vi "Velocity Acceleration.vi"() -> ()   [LabVIEW 2024]
panel:
  out "String":string
  out "Acceleration":dbl[](array[numeric])
  out "Velocity":dbl[](array[numeric])
  in  "DIsplacement":dbl[](array[numeric])
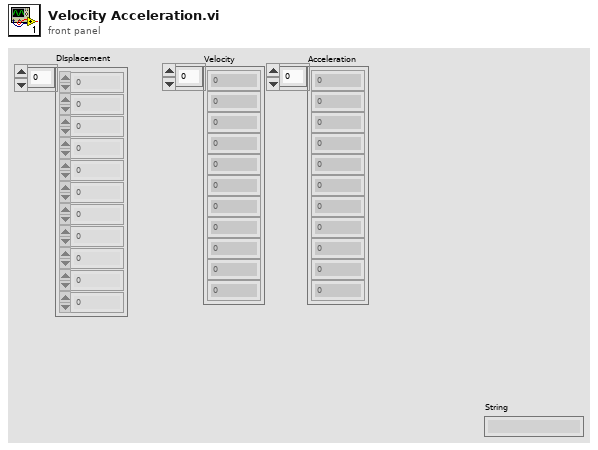
[diagram p1: front panel]
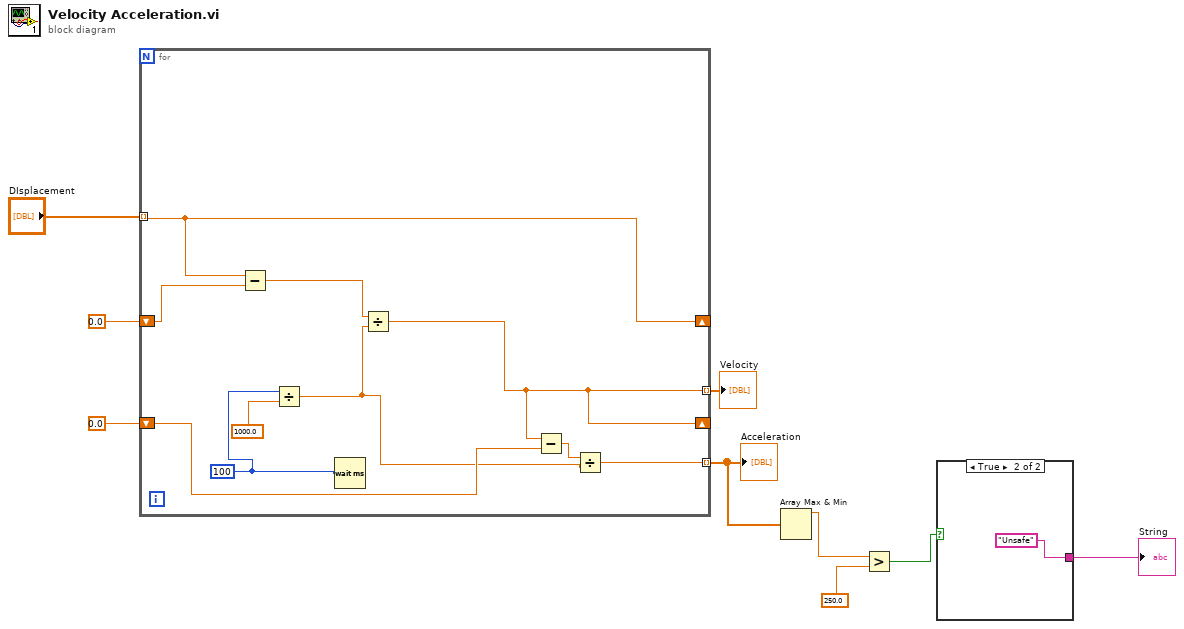
[diagram p0: block diagram]
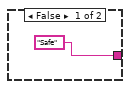
[diagram p2: hidden frame]
diagram:
  n1 = for {
    tunnel: "DIsplacement" -> [w17] mode=indexing
    shift-right: [w17] -> _
    shift-left: 0.0 ("Numeric") -> [w16]
    tunnel: [w13] -> w7 mode=indexing
    shift-right: [w13] -> _
    shift-left: 0.0 -> [w14]
    tunnel: [w10] -> w5 mode=indexing
    w18 = u32 100 ("milliseconds to wait")
    n2 = Subtract(x=w17, y=w16) -> (x-y=w15:dbl)
    n3 = Divide(x=w18, y=1000.0) -> (x/y=w11:dbl)
    n4 = Wait (ms)(milliseconds to wait=w18) -> ()  [unwired: 1 out]
    n5 = Divide(x=w15, y=w11) -> (x/y=w13:dbl)
    n6 = Subtract(x=w13, y=w14) -> (x-y=w12:dbl)
    n7 = Divide(x=w12, y=w11) -> (x/y=w10:dbl)
  }
  "Velocity" <- w7
  "Acceleration" <- w5
  n8 = Array Max & Min(array=w5) -> (max value=w3:dbl)  [unwired: 3 out]
  n9 = Greater?(x=w3, y=250.0) -> (0:w1:bool)
  n10 = case shown="True" w1 {
    tunnel: ["Safe" "Unsafe"] -> w2
    frame False {
    }
    frame True {
    }
  }
  "String" <- w2
